vi "Create.vi"(7 "mode settings":variant, 8 "error in":errorcluster, 9 "number of default channels":i32, 10 "channel settings":variant, 11 "digital input and output mode in":refnum<class "Digital Input and Output Mode.lvclass">) -> (0 "error out":errorcluster, 1 "channels":refnum<class "Channel.lvclass">[](array[class]), 3 "digital input and output mode out":refnum<class "Digital Input and Output Mode.lvclass">)   [LabVIEW 2020, in "Scan Engine Scripting.lvlib" / "Digital Input and Output Mode.lvclass"]
uses:
  Digital Input and Output Mode.lvclass
  Channel Classes/Channel/Channel.lvclass
  Digital Output Mode/Digital Output Mode.lvclass
  Digital Input Mode/Digital Input Mode.lvclass
  Controls/digital channel settings.ctl
  Scan Engine Scripting.lvlib
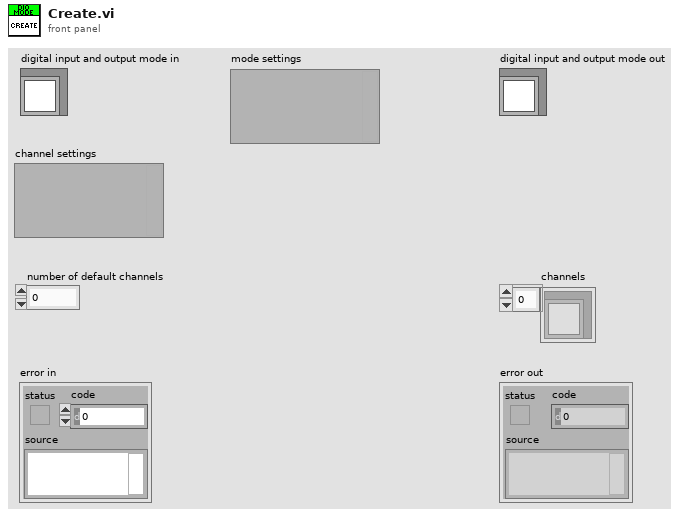
[diagram p1: front panel]
types:
  T1 = typedef "Scan Engine Scripting.lvlib/digital channel settings.ctl" = cluster{"name":string, "default value":bool}
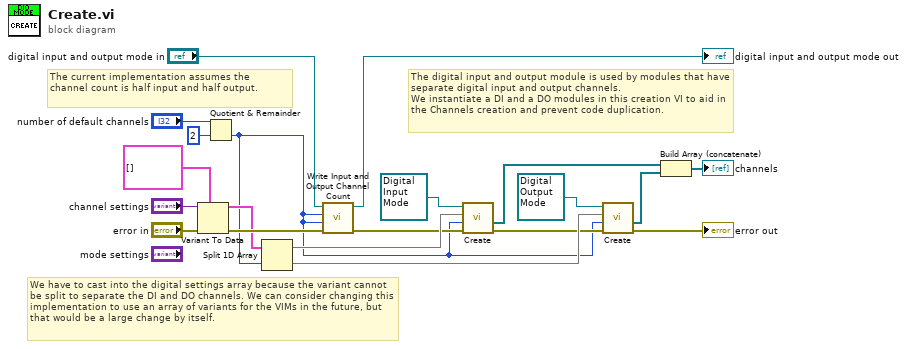
[diagram p0: block diagram]
diagram:
  # "We have to cast into the digital settings array because the variant cannot be split to separate the DI and DO channels. We can consider changing this implementation to use an array of variants for the VIMs in the future, but that would be a large change by itself."
  # "The current implementation assumes the channel count is half input and half output."
  # "The digital input and output module is used by modules that have separate digital input and output channels.\nWe instantiate a DI and a DO modules in this creation VI to aid in the Channels creation and prevent code duplication."
  n1 = Variant To Data(error in="error in", type=T1[] [] ("channel settings"), Variant="channel settings") -> (data=w2:T1[], error out=w4:errorcluster)
  n2 = Quotient & Remainder(x="number of default channels", y=2) -> (floor(x/y)=w1:i32)  [unwired: 1 out]
  n3 = Split 1D Array(array=w2, index=w1) -> (first subarray=w20:T1[], second subarray=w19:T1[])
  n4 = call "Write Input and Output Channel Count.vi"("error in"=w4, "number output channels"=w1, "number input channels"=w1, "digital input and output mode in"="digital input and output mode in") -> ("error out"=w7:errorcluster, "digital input and output mode out"=→"digital input and output mode out":refnum<class "Digital Input and Output Mode.lvclass">)  [unwired: 6 in]
  n5 = call-dynamic "Create.vi"("error in"=w7, "number of default channels"=w1, "channel settings"=w20, "digital input mode in"=refnum<class "Digital Input Mode.lvclass"> refnum ("Scan Engine Scripting.lvlib:Digital Input Mode.lvclass")) -> ("error out"=w12:errorcluster, "channels"=w15:refnum<class "Channel.lvclass">[])  [unwired: 5 in, 1 out]
  n6 = call-dynamic "Create.vi"("error in"=w12, "number of default channels"=w1, "channel settings"=w19, "digital output mode in"=refnum<class "Digital Output Mode.lvclass"> refnum ("Scan Engine Scripting.lvlib:Digital Output Mode.lvclass")) -> ("error out"=→"error out":errorcluster, "channels"=w14:refnum<class "Channel.lvclass">[])  [unwired: 5 in, 1 out]
  n7 = Build Array (concatenate)(w15, w14) -> (→"channels":refnum<class "Channel.lvclass">[])
